vi "NF LI56xx dvr qQUEStionable.vi"(8 "error in":errorcluster caption="error in (no error)" {"code" format="%.0x"}, 11 "VISA resource name":refnum<visa-resource-name>) -> (0 "error out":errorcluster {"code" format="%.0x"}, 2 "query the Questionable Event register":string, 3 "VISA resource name copy":refnum<visa-resource-name>)   [LabVIEW 2019]
doc: "Queries the Questionable Event register (QUER)."
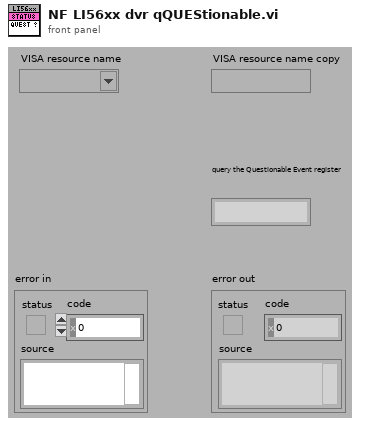
[diagram p1: front panel]
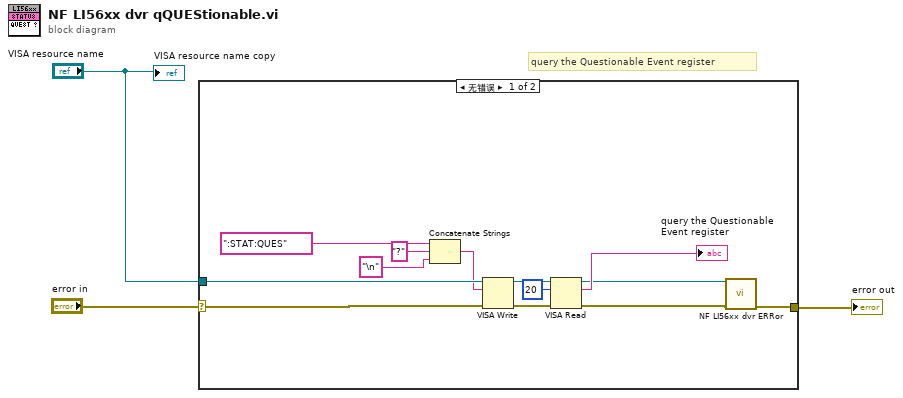
[diagram p0: block diagram]
diagram:
  # "query the Questionable Event register"
  n1 = case shown="无错误" "error in" {
    selector: "error in" -> [w16 w17]
    tunnel: [w11 w17] -> w3
    tunnel: "VISA resource name" -> [w15 _]
    frame No Error {
      n2 = Concatenate Strings(":STAT:QUES" ("•¶Žš—ñ"), "?" ("Œ`Ž®•¶Žš—ñ"), "\n" ("Œ`Ž®•¶Žš—ñ")) -> (w5:string)
      n3 = VISA Write(VISA resource name=w15, write buffer=w5, error in (no error)=w16) -> (VISA resource name out=w8:refnum<visa-resource-name>, error out=w9:errorcluster)  [unwired: 1 out]
      n4 = VISA Read(VISA resource name=w8, byte count=u32 20 ("バイトカウント（0）"), error in (no error)=w9) -> (VISA resource name out=w13:refnum<visa-resource-name>, read buffer=→"query the Questionable Event register":string, error out=w12:errorcluster)  [unwired: 1 out]
      n5 = call "NF LI56xx dvr ERRor.vi"("VISA resource name"=w13, "error in (no error)"=w12) -> ("error out"=w11:errorcluster)  [unwired: 10 in, 3 out]
    }
    frame Error {
    }
  }
  "error out" <- w3
  "VISA resource name copy" <- "VISA resource name"
